vi "Inst.RP100.setStrain.vi"(8 "error in (no error)":errorcluster, 10 "data in":variant, 11 "Inst.RP100 in":refnum<class "Inst.RP100.lvclass">) -> (0 "error out":errorcluster, 3 "Inst.RP100 out":refnum<class "Inst.RP100.lvclass">)   [LabVIEW 2019, in "Inst.RP100.lvclass"]
uses:
  Inst.RP100.lvclass
  Typedefs/Output Channel--Enum.ctl
  Typedefs/Output State--Enum.ctl
  Typedefs/SetStrain--Cluster.ctl
  Inst.RP100.lvclass/Inst.RP100.ctl
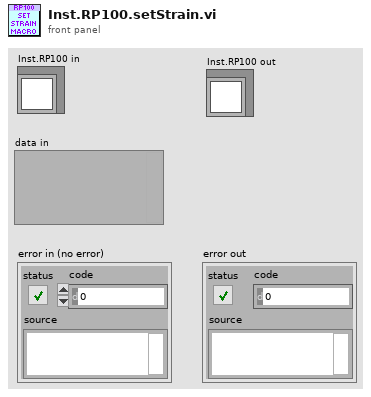
[diagram p1: front panel]
types:
  T1 = typedef "Inst.RP100.lvclass/SetStrain--Cluster.ctl" = cluster{"Strain (V)":dbl, "Slew (V/s)":dbl}
  T2 = typedef "Inst.RP100.lvclass/Output Channel--Enum.ctl" = enum16{"Output 1", "Output 2"}
  T3 = typedef "Inst.RP100.lvclass/Output State--Enum.ctl" = enum16{"Shorted", "Enabled"}
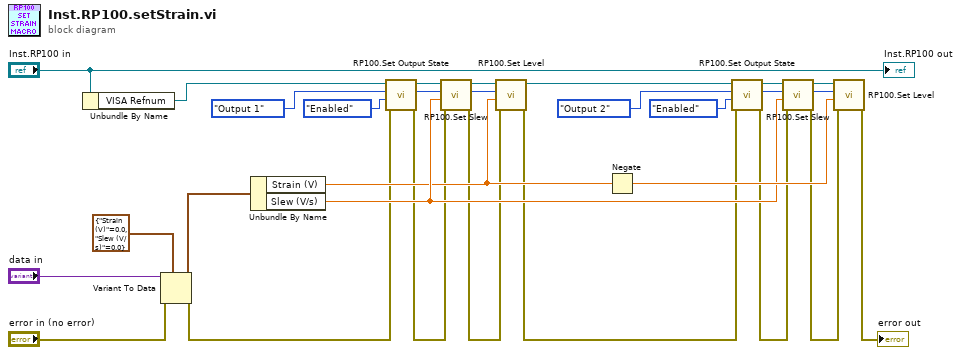
[diagram p0: block diagram]
diagram:
  n1 = Unbundle By Name("Inst.RP100 in") -> ("VISA Refnum"=w4:refnum<visa-resource-name>)
  n2 = Variant To Data(error in="error in (no error)", type=T1 {"Strain (V)"=0.0, "Slew (V/s)"=0.0} ("Data in"), Variant="data in") -> (data=w7:T1, error out=w5:errorcluster)
  n3 = Unbundle By Name(w7) -> ("Strain (V)"=w17:dbl, "Slew (V/s)"=w24:dbl)
  n4 = call "RP100.Set Output State.vi"("error in (no error)"=w5, "Output State"=Output_State--Enum."Enabled", "Output Channel"=Output_Channel--Enum."Output 1", "VISA resource name"=w4) -> ("error out"=w11:errorcluster, "Output Channel"=w19:T2, "VISA Refnum out"=w18:refnum<visa-resource-name>)  [unwired: 5 in]
  n5 = call "RP100.Set Slew.vi"("error in (no error)"=w11, "Slew (V/s)"=w24, "Output Channel"=w19, "VISA resource name"=w18) -> ("error out"=w12:errorcluster, "Output Channel"=w20:T2, "VISA Refnum out"=w21:refnum<visa-resource-name>)  [unwired: 5 in]
  n6 = call "RP100.Set Level.vi"("error in (no error)"=w12, "Level (V)"=w17, "Output Channel"=w20, "VISA resource name"=w21) -> ("error out"=w13:errorcluster, "VISA Refnum out"=w22:refnum<visa-resource-name>)  [unwired: 5 in, 1 out]
  n7 = Negate(x=w17) -> (-x=w25:dbl)
  n8 = call "RP100.Set Output State.vi"("error in (no error)"=w13, "Output State"=Output_State--Enum."Enabled", "Output Channel"=Output_Channel--Enum."Output 2", "VISA resource name"=w22) -> ("error out"=w14:errorcluster, "Output Channel"=w23:T2, "VISA Refnum out"=w28:refnum<visa-resource-name>)  [unwired: 5 in]
  n9 = call "RP100.Set Slew.vi"("error in (no error)"=w14, "Slew (V/s)"=w24, "Output Channel"=w23, "VISA resource name"=w28) -> ("error out"=w15:errorcluster, "Output Channel"=w26:T2, "VISA Refnum out"=w27:refnum<visa-resource-name>)  [unwired: 5 in]
  n10 = call "RP100.Set Level.vi"("error in (no error)"=w15, "Level (V)"=w25, "Output Channel"=w26, "VISA resource name"=w27) -> ("error out"=→"error out":errorcluster)  [unwired: 5 in, 2 out]
  "Inst.RP100 out" <- "Inst.RP100 in"
